vi "HTTP-Init.vi"(8 "error in (no error)":errorcluster, 11 "ByteGSWebAPI-V0 in":refnum<class "ByteGSWebAPI-V0.lvclass">) -> (0 "error out":errorcluster, 3 "ByteGSWebAPI-V0 out":refnum<class "ByteGSWebAPI-V0.lvclass">)   [LabVIEW 2019, in "ByteGSWebAPI.lvlib" / "ByteGSWebAPI-V0.lvclass"]
doc: "Apre una nuova connessione HTTP e setta il content type a \"application/json\""
uses:
  ByteGSWebAPI-V0.lvclass
  ByteGSWebAPI-V0.lvclass/ByteGSWebAPI-V0.ctl
  <vilib>/httpClient/LabVIEWHTTPClient.lvlib
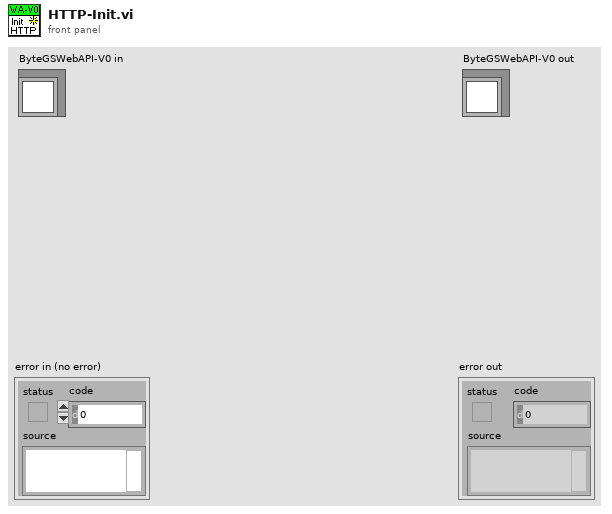
[diagram p1: front panel]
types:
  T1 = typedef "LabVIEWHTTPClient.lvlib/ClientHandle.ctl" = refnum<k1>
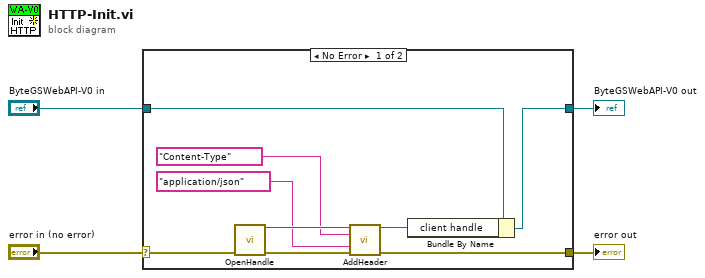
[diagram p0: block diagram]
diagram:
  n1 = case shown="No Error" "error in (no error)" {
    selector: "error in (no error)" -> [w6 w15]
    tunnel: [w5 w15] -> w3
    tunnel: [w8 w14] -> w1
    tunnel: "ByteGSWebAPI-V0 in" -> [w13 w14]
    frame No Error {
      n2 = call <vilib>:"OpenHandle.vi"("error in (no error)"=w6) -> ("client handle out"=w11:T1, "error out"=w12:errorcluster)  [unwired: 13 in]
      n3 = call <vilib>:"AddHeader.vi"("client handle"=w11, "header"="Content-Type", "value"="application/json", "error in (no error)"=w12) -> ("client handle out"=w7:T1, "error out"=w5:errorcluster)  [unwired: 10 in]
      n4 = Bundle By Name(cluster=w13, "client handle"=w7) -> (w8:refnum<class "ByteGSWebAPI-V0.lvclass">)
    }
    frame Error {
    }
  }
  "error out" <- w3
  "ByteGSWebAPI-V0 out" <- w1
